vi "IsEquivalentI16.vi"(4 "Y":i16, 5 "X":i16) -> (1 "Equivalent?":bool)   [LabVIEW 2017, in "GPComparison.lvlib"]
doc: "<B>X</B> and <B>Y</B> are <B>Equivalent?</B> only if they are strictly equal (since they are well-defined integers).\n\nThis VI is inlined.\n\nSteen Schmidt\nGPower\n22/10 2016"
uses:
  GPComparison.lvlib
panel:
  # "Copyright © 2016\nGPower\nSee enclosed license file for terms and conditions"
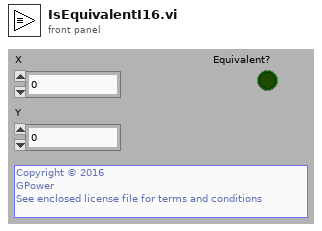
[diagram p1: front panel]
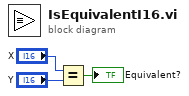
[diagram p0: block diagram]
diagram:
  n1 = Equal?(x="X", y="Y") -> (x = y?=→"Equivalent?":bool)
